vi "SwerveOdometry_NewZeroCenter.vi"(11 "gyroAngle":T4={"VALUE"=0.0, "COS"=1.0, "SIN"=0.0} {"SIN" format="%13.4f"; "COS" format="%13.4f"; "VALUE" format="%13.4f"}) -> (3 "SWERVE_DRIVE_ODOMETRY":T1={"POSE"={"TRANSLATION"={"X"=0.0, "Y"=0.0}, "ROTATION"={"VALUE"=0.0, "COS"=1.0, "SIN"=0.0}}, "GyroOffset"={"VALUE"=0.0, "COS"=1.0, "SIN"=0.0}, "PreviousAngle"={"VALUE"=0.0, "COS"=1.0, "SIN"=0.0}, "PrevTime"=0.0} {"PreviousAngle"."SIN" format="%13.4f"; "PreviousAngle"."COS" format="%13.4f"; "PreviousAngle"."VALUE" format="%13.4f"; "GyroOffset"."SIN" format="%13.4f"; "GyroOffset"."COS" format="%13.4f"; "GyroOffset"."VALUE" format="%13.4f"; "POSE"."ROTATION"."SIN" format="%13.4f"; "POSE"."ROTATION"."COS" format="%13.4f"; "POSE"."ROTATION"."VALUE" format="%13.4f"; "POSE"."TRANSLATION"."Y" format="%14.3f"; "POSE"."TRANSLATION"."X" format="%14.3f"})   [LabVIEW 2019, in "Trajectory_Library.lvlib"]
doc: "Constructs a SwerveDriveOdometry object with the default pose at the origin.\n \nParameters:\n - gyroAngle - The angle reported by the gyroscope.\n\nReturns:\n - SwerveDriveOdometry - Data Structure"
uses:
  Trajectory_Library.lvlib
  TypeDef/ROTATION2D.ctl
  TypeDef/SWERVE_DRIVE_ODOMETRY.ctl
  TypeDef/POSE2D.ctl
  TypeDef/TRANSLATION2D.ctl
  Rotation2d_CreateAngle.vi
  Translation2d_Create.vi
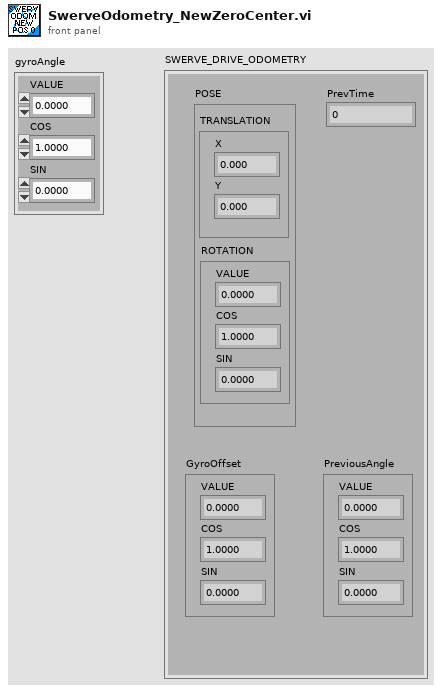
[diagram p1: front panel]
types:
  T1 = typedef "Trajectory_Library.lvlib/SWERVE_DRIVE_ODOMETRY.ctl" = cluster{"POSE":T2, "GyroOffset":T4, "PreviousAngle":T4, "PrevTime":dbl}
  T2 = typedef "Trajectory_Library.lvlib/POSE2D.ctl" = cluster{"TRANSLATION":T3, "ROTATION":T4}
  T3 = typedef "Trajectory_Library.lvlib/TRANSLATION2D.ctl" = cluster{"X":dbl, "Y":dbl}
  T4 = typedef "Trajectory_Library.lvlib/ROTATION2D.ctl" = cluster{"VALUE":dbl, "COS":dbl, "SIN":dbl}
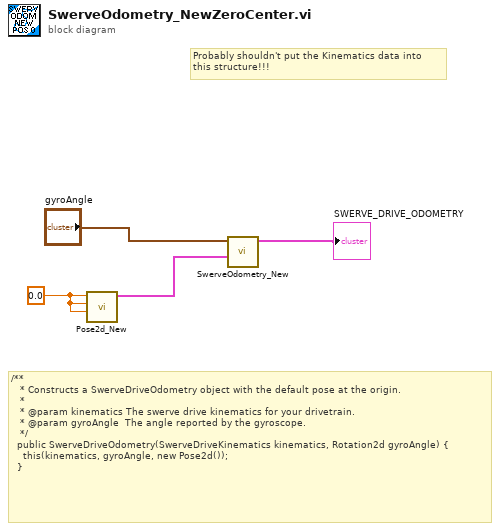
[diagram p0: block diagram]
diagram:
  w3 = 0.0 ("X")
  # "Probably shouldn't put the Kinematics data into\nthis structure!!!"
  # "/**\n   * Constructs a SwerveDriveOdometry object with the default pose at the origin.\n   *\n   * @param kinematics The swerve drive kinematics for your drivetrain.\n   * @param gyroAngle  The angle reported by the gyroscope.\n   */\n  public SwerveDriveOdometry(SwerveDriveKinematics kinematics, Rotation2d gyroAngle) {\n    this(kinematics, gyroAngle, new Pose2d());\n  }"
  n1 = call "Pose2d_New.vi"("Heading"=w3, "Y"=w3, "X"=w3) -> ("out POSe"=w2:T2)  [unwired: 8 in]
  n2 = call "SwerveOdometry_New.vi"("InitialPose"=w2, "gyroAngle"="gyroAngle") -> ("SWERVE_DRIVE_ODOMETRY"=→"SWERVE_DRIVE_ODOMETRY":T1)  [unwired: 9 in]
